vi "Find all incomplete calcs.vi"() -> ()   [LabVIEW 2010]
panel:
  out "Excel Table":string
  out "Folder Path":path
  out "Table Control":string[][](table)
  in  "Source Directory":path=path "D:/Ab-initio/VASP Calcs/2D_Grain Boundaries/Batch18_20130828/A3B12_Periodic_Twin/CONTCAR"
  # "Calc Time"
  # "dE"
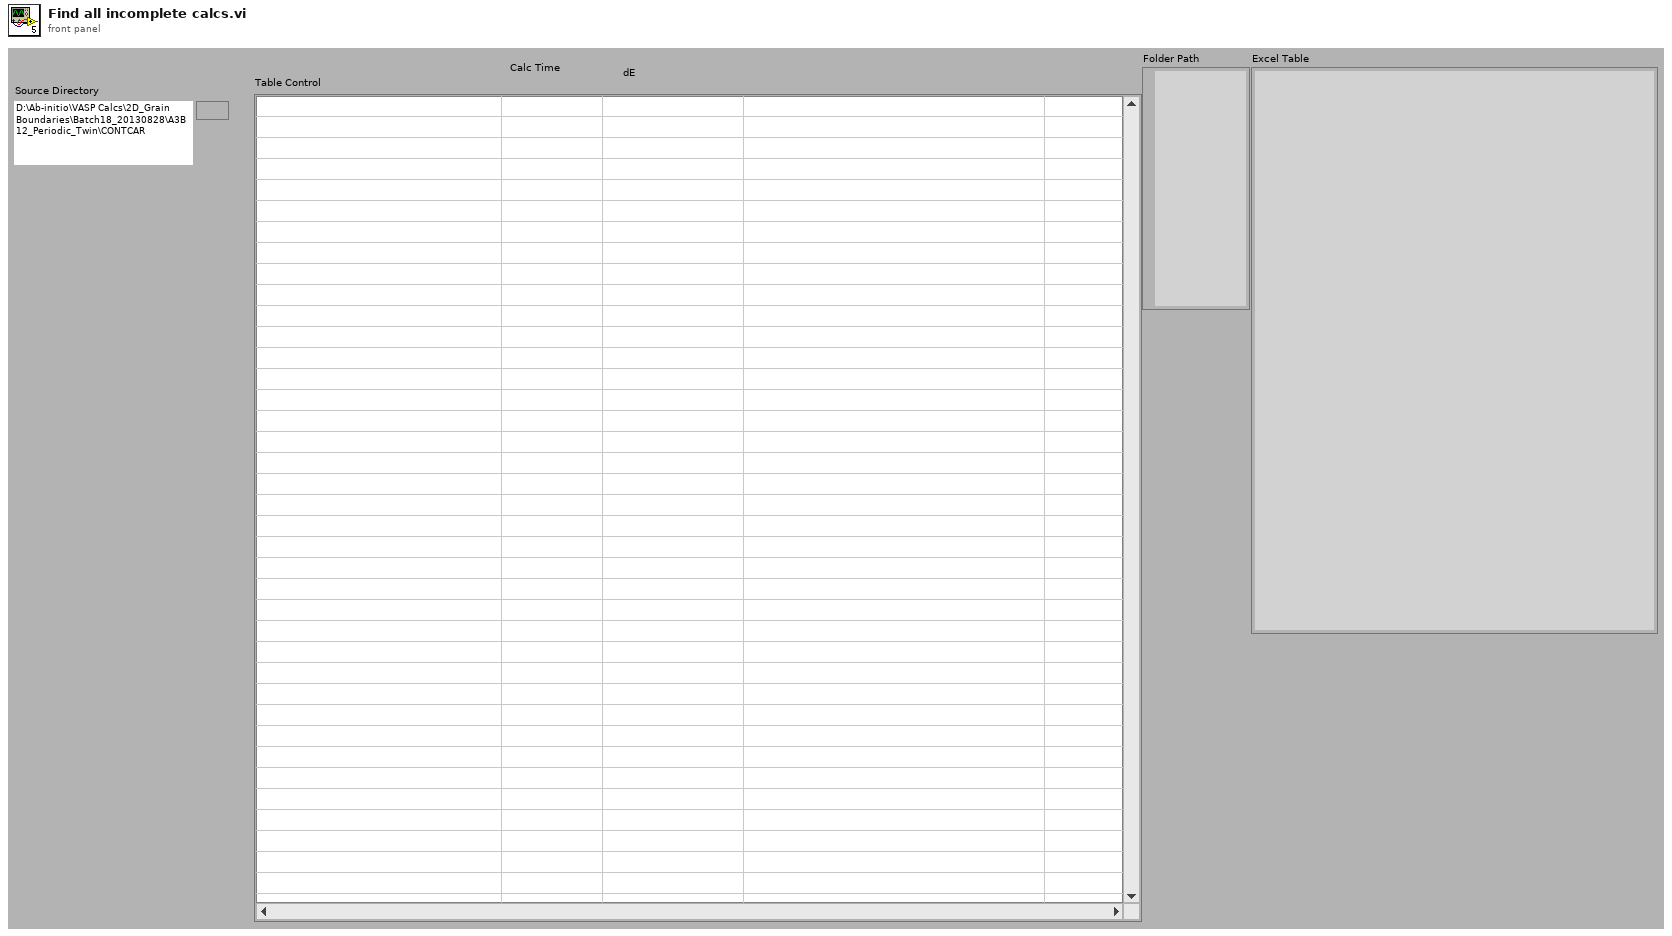
[diagram p1: front panel]
types:
  T1 = cluster{"INCAR ID":string, "IBRION":string, "ISIF":string, "ISMEAR":string, "ISPIN":string, "Net Charge":i32}
  T2 = cluster{"OSZICAR data":cluster{"Total Free Energy (eV)":dbl, "E0 at Sigma=0 (eV)":dbl, "dE (eV)":dbl, "Electronic Relaxation":dbl[][]}[], "Ionic Relaxation Energies Array (eV)":dbl[], "Bulk Formation Energies Array (eV)":dbl[]}
  T3 = cluster{"Total Free Energy (eV)":dbl, "E0 at Sigma=0 (eV)":dbl, "dE (eV)":dbl, "Electronic Relaxation":dbl[][]}[]
  T4 = cluster{"Total Free Energy (eV)":dbl, "E0 at Sigma=0 (eV)":dbl, "dE (eV)":dbl, "Electronic Relaxation":dbl[][]}
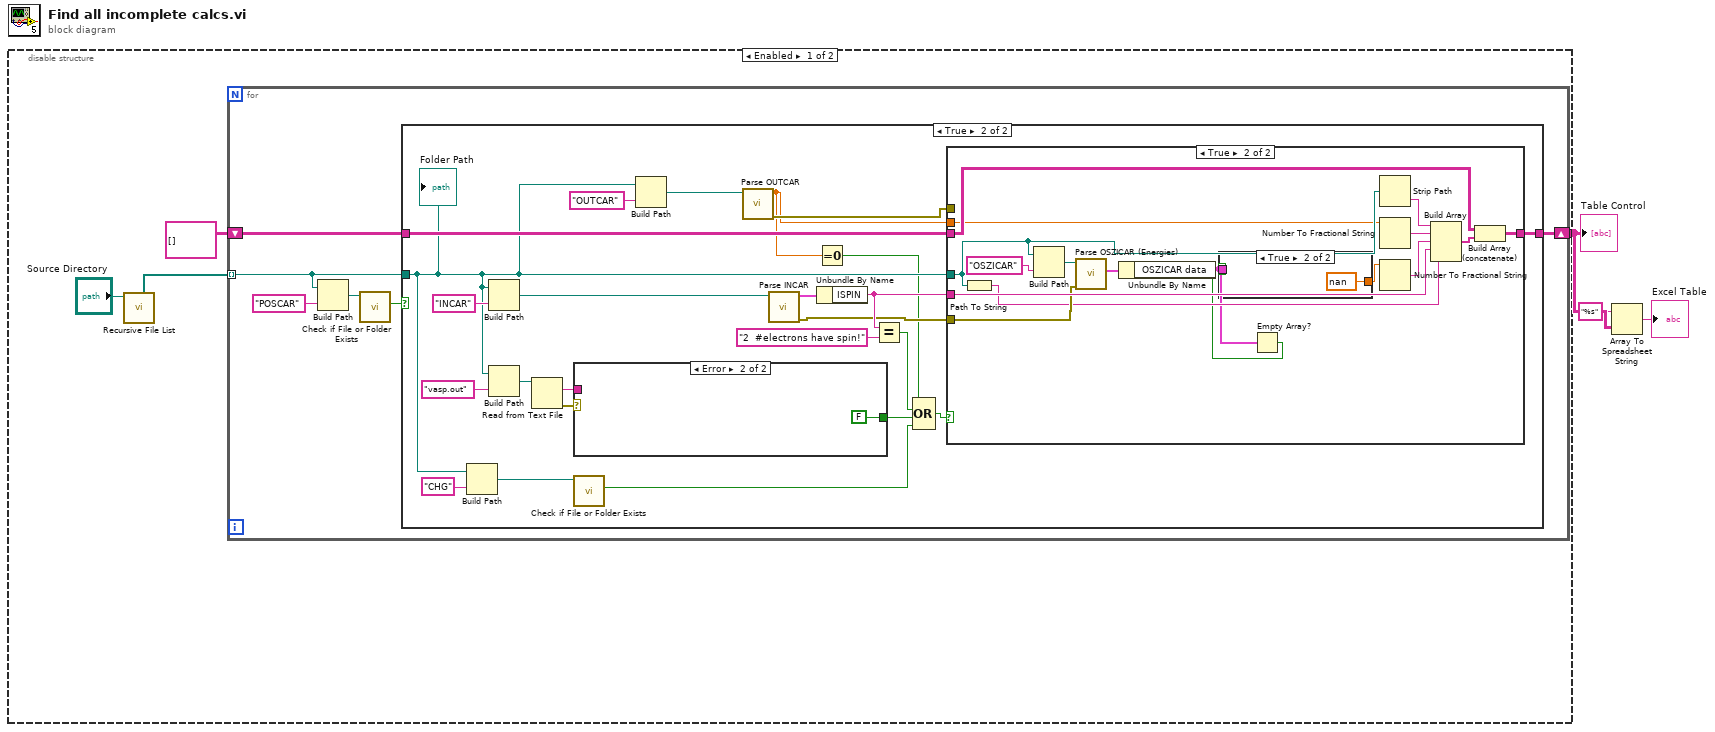
[diagram p0: block diagram]
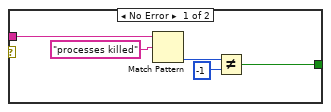
[diagram p3: hidden frame]
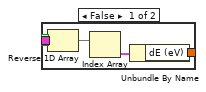
[diagram p5: hidden frame]
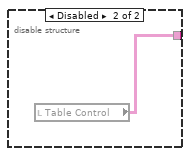
[diagram p6: hidden frame]
diagram:
  n1 = disable-structure shown="Enabled" {
    disable-tunnel: [w4 w68] -> w3
    frame Enabled {
      n2 = call <vilib>:"Recursive File List.vi"("Folder Path"="Source Directory") -> ("All Folders"=w6:path[])  [unwired: 6 in, 4 out]
      n3 = for {
        tunnel: w6 -> [w10] mode=indexing
        shift-right: [w9] -> w4
        shift-left: string[][] [] -> [w8]
        n4 = Build Path(base path=w10, name or relative path="POSCAR" ("pattern")) -> (appended path=w12:path)
        n5 = call <vilib>:"Check if File or Folder Exists.vi"("path"=w12) -> ("file or folder exists?"=w11:bool)  [unwired: 8 in, 2 out]
        n6 = case shown="True" w11 {
          tunnel: w10 -> [_ w18]
          tunnel: [w14 w30] -> w9
          tunnel: w8 -> [w14 w29]
          frame False {
          }
          frame True {
            n7 = Build Path(base path=w18, name or relative path="CHG") -> (appended path=w34:path)
            n8 = Build Path(base path=w18, name or relative path="INCAR") -> (appended path=w24:path)
            n9 = Build Path(base path=w18, name or relative path="vasp.out") -> (appended path=w37:path)
            n10 = Read from Text File(file (use dialog)=w37) -> (text=w38:string, error out=w28:errorcluster)  [unwired: 3 in, 2 out]
            n11 = case shown="Error" w28 {
              tunnel: w38 -> [w42 _]
              tunnel: [w39 FALSE] -> w32
              frame No Error {
                n12 = Match Pattern(string=w42, regular expression="processes killed") -> (offset past match=w41:i32)  [unwired: 1 in, 3 out]
                n13 = Not Equal?(x=w41, y=-1) -> (x != y?=w39:bool)
              }
              frame Error {
              }
            }
            n14 = call <vilib>:"Check if File or Folder Exists.vi"("path"=w34) -> ("file or folder exists?"=w33:bool)  [unwired: 8 in, 2 out]
            n15 = Build Path(base path=w18, name or relative path="OUTCAR") -> (appended path=w20:path)
            n16 = call "Parse OUTCAR.vi"("OUTCAR File"=w20) -> ("error out"=w17:errorcluster, "Calc Time (Hrs)"=w16:dbl)  [unwired: 8 in, 1 out]
            n17 = call "Parse INCAR.vi"("INCAR File"=w24) -> ("error out"=w21:errorcluster, "INCAR Summary"=w27:T1)  [unwired: 6 in, 3 out]
            n18 = Equal To 0?(x=w16) -> (x = 0?=w15:bool)
            n19 = Unbundle By Name(w27) -> ("ISPIN"=w22:string)
            n20 = Equal?(x=w22, y="2  #electrons have spin!") -> (x = y?=w25:bool)
            n21 = Compound Arithmetic op=OR(w15, w25, w32, w33) -> (w31:bool)
            n22 = case shown="True" w31 {
              tunnel: w18 -> [_ w58]
              tunnel: [w45 w59] -> w30
              tunnel: w29 -> [w45 w61]
              tunnel: w22 -> [_ w52]
              tunnel: w21 -> [_ w51]
              tunnel: w16 -> [_ w49]
              tunnel: w17 -> [_ _]
              frame False {
              }
              frame True {
                n23 = Path To String(path=w58) -> (string=w50:string)
                n24 = Build Path(base path=w58, name or relative path="OSZICAR") -> (appended path=w57:path)
                n25 = call "Parse OSZICAR (Energies).vi"("error in (no error)"=w51, "OSZICAR File"=w57) -> ("OSZICAR Raw"=w55:T2)  [unwired: 6 in, 3 out]
                n26 = Unbundle By Name(w55) -> ("OSZICAR data"=w47:T3)
                n27 = Empty Array?(array=w47) -> (empty?=w46:bool)
                n28 = case shown="True" w46 {
                  tunnel: [w64 nan ("dE (eV)")] -> w48
                  tunnel: w47 -> [w63 _]
                  frame False {
                    n29 = Reverse 1D Array(array=w63) -> (reversed array=w66:T3)
                    n30 = Index Array(array=w66) -> (element=w65:T4)  [unwired: 1 in]
                    n31 = Unbundle By Name(w65) -> ("dE (eV)"=w64:dbl)
                  }
                  frame True {
                  }
                }
                n32 = Strip Path(path=w58) -> (name=w62:string)  [unwired: 1 out]
                n33 = Number To Fractional String(number=w49) -> (F-format string=w54:string)  [unwired: 3 in]
                n34 = Number To Fractional String(number=w48) -> (F-format string=w53:string)  [unwired: 3 in]
                n35 = Build Array(w62, w54, w53, w52, w50) -> (w60:string[])
                n36 = Build Array (concatenate)(w61, w60) -> (w59:string[][])
              }
            }
            "Folder Path" <- w18
          }
        }
      }
    }
    frame Disabled {
      n37 = local read "Table Control"() -> (w68:string[][])
    }
  }
  "Table Control" <- w3
  n38 = Array To Spreadsheet String(array=w3, 3:"%s" ("format string")) -> (spreadsheet string=→"Excel Table":string)  [unwired: 1 in]
